vi "Read.vi"(8 "error in (no error)":errorcluster, 11 "TDMS File in":refnum<class "File.lvclass">) -> (0 "error out":errorcluster, 1 "File Properties":refnum<class "Variant.lvclass">, 2 "Groups":refnum<class "Group.lvclass">[](array[class]), 3 "File Path":path)   [LabVIEW 2020, in "TDMS.lvlib" / "File.lvclass"]
doc: "Read File Path, Groups and File Properties."
uses:
  File.lvclass
  TDMS Group/Group.lvclass
  PPL/HDH.Data.Generic.lvlibp/Generic Data/Variant/Variant.lvclass
  File.lvclass/File.ctl
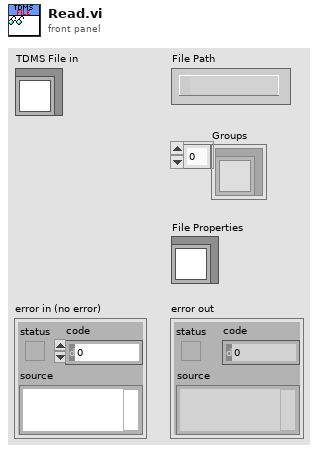
[diagram p1: front panel]
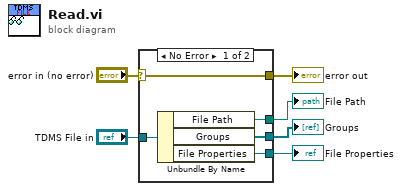
[diagram p0: block diagram]
diagram:
  n1 = case shown="No Error" "error in (no error)" {
    selector: "error in (no error)" -> [w11 w12]
    tunnel: [w11 w12] -> w5
    tunnel: "TDMS File in" -> [w10 _]
    tunnel: [w9 _] -> w3
    tunnel: [w8 _] -> w2
    tunnel: [w7 _] -> w1
    frame No Error {
      n2 = Unbundle By Name(w10) -> ("File Path"=w9:path, "Groups"=w8:refnum<class "Group.lvclass">[], "File Properties"=w7:refnum<class "Variant.lvclass">)
    }
    frame Error {
    }
  }
  "error out" <- w5
  "File Path" <- w3
  "Groups" <- w2
  "File Properties" <- w1
